vi "UpdateChanged.vi"(10 "WorldMapEdge":T1, 11 "RVCLibrary_Bug in":refnum<class "RVCLibrary_Bug2.lvclass">) -> (2 "updated":bool, 3 "RVCLibrary_Bug2 out":refnum<class "RVCLibrary_Bug2.lvclass">)   [LabVIEW 2013, in "RVCLibrary_Bug2.lvclass"]
uses:
  RVCLibrary_Bug2.lvclass
  <vilib>/robotics/Navigation/shared/MapNode/AbstractMapNode/NI_Robotics_AbstractMapNode.lvclass
  <vilib>/robotics/Navigation/shared/MapNode/AbstractDstarNode/NI_Robotics_AbstractDstarNode.lvclass
  <vilib>/robotics/Navigation/shared/WorldMap/World Map Edge.ctl
  <vilib>/robotics/Navigation/shared/WorldMap/AbstractWorldMap/NI_Robotics_AbstractWorldMap.lvclass
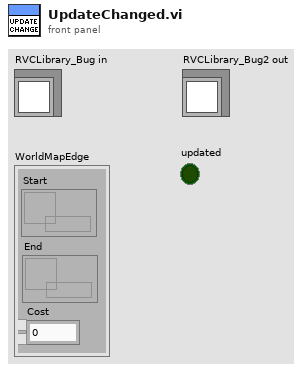
[diagram p1: front panel]
types:
  T1 = typedef "NI_Robotics_AbstractWorldMap.lvclass/World Map Edge.ctl" = cluster{"Start":refnum<data-value>, "End":refnum<data-value>, "Cost":dbl}
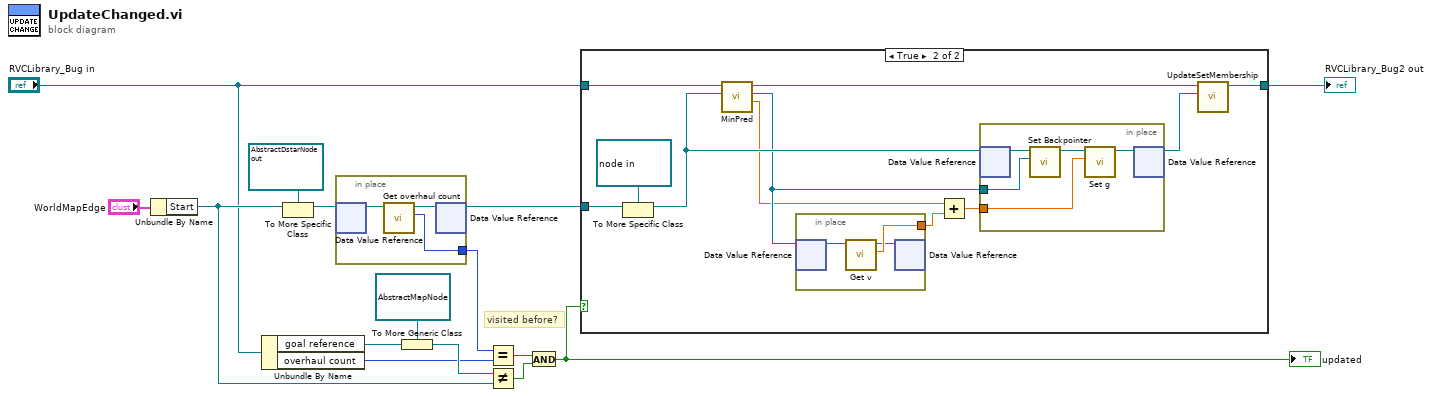
[diagram p0: block diagram]
diagram:
  # "visited before?"
  n1 = Unbundle By Name("WorldMapEdge") -> ("Start"=w10:refnum<data-value>)
  n2 = Unbundle By Name("RVCLibrary_Bug in") -> ("goal reference"=w9:refnum<data-value>, "overhaul count"=w7:i32)
  n3 = To More Specific Class(target class=refnum<data-value> refnum ("data value reference"), reference=w10) -> (specific class reference=w5:refnum<data-value>)  [unwired: 1 in, 1 out]
  n4 = in-place {
    in-place-border: [w18] -> w8
    n5 = in-place-dvr #1(w5) -> (w17:refnum<class "NI_Robotics_AbstractDstarNode.lvclass">)  [unwired: 1 out]
    n6 = call <vilib>:"Get overhaul count.vi"("AbstractDstarNode in"=w17) -> ("overhaul count"=w18:i32, "AbstractDstarNode out"=w16:refnum<class "NI_Robotics_AbstractDstarNode.lvclass">)  [unwired: 9 in]
    n7 = in-place-dvr #1(w16) -> (w4:refnum<data-value>)  [unwired: 1 out]
  }
  n8 = To More Generic Class(target class=refnum<data-value> refnum ("Start"), reference=w9) -> (generic class reference=w14:refnum<data-value>)
  n9 = Equal?(x=w8, y=w7) -> (x = y?=w6:bool)
  n10 = Not Equal?(x=w14, y=w10) -> (x != y?=w12:bool)
  n11 = And(x=w6, y=w12) -> (x .and. y?=w3:bool)
  "updated" <- w3
  n12 = case shown="True" w3 {
    tunnel: "RVCLibrary_Bug in" -> [w19 w20]
    tunnel: w4 -> [_ w25]
    tunnel: [w19 w27] -> w1
    frame False {
    }
    frame True {
      n13 = To More Specific Class(target class=refnum<data-value> refnum ("node ref in"), reference=w25) -> (specific class reference=w30:refnum<data-value>)  [unwired: 1 in, 1 out]
      n14 = call "MinPred.vi"("node ref in"=w30, "RVCLibrary_Bug in"=w20) -> ("cost of node to min pred"=w22:dbl, "min node ref"=w24:refnum<data-value>, "RVCLibrary_Bug out"=w28:refnum<class "RVCLibrary_Bug2.lvclass">)  [unwired: 6 in, 1 out]
      n15 = in-place {
        in-place-border: [w33] -> w23
        n16 = in-place-dvr #2(w24) -> (w32:refnum<class "NI_Robotics_AbstractDstarNode.lvclass">)  [unwired: 1 out]
        n17 = call <vilib>:"Get v.vi"("AbstractDstarNode in"=w32) -> ("v"=w33:dbl, "AbstractDstarNode out"=w31:refnum<class "NI_Robotics_AbstractDstarNode.lvclass">)  [unwired: 9 in]
        n18 = in-place-dvr #2(w31) -> ()  [unwired: 2 out]
      }
      n19 = Add(x=w22, y=w23) -> (x+y=w21:dbl)
      n20 = in-place {
        in-place-border: w24 -> [w38]
        in-place-border: w21 -> [w34]
        n21 = in-place-dvr #3(w30) -> (w37:refnum<class "NI_Robotics_AbstractDstarNode.lvclass">)  [unwired: 1 out]
        n22 = call <vilib>:"Set Backpointer.vi"("BackPointer"=w38, "AbstractDstarNode in"=w37) -> ("AbstractDstarNode out"=w36:refnum<class "NI_Robotics_AbstractDstarNode.lvclass">)  [unwired: 8 in, 1 out]
        n23 = call <vilib>:"Set g.vi"("g"=w34, "AbstractDstarNode in"=w36) -> ("AbstractDstarNode out"=w35:refnum<class "NI_Robotics_AbstractDstarNode.lvclass">)  [unwired: 9 in]
        n24 = in-place-dvr #3(w35) -> (w29:refnum<data-value>)  [unwired: 1 out]
      }
      n25 = call "UpdateSetMembership.vi"("node ref in"=w29, "RVCLibrary_Bug in"=w28) -> ("RVCLibrary_Bug out"=w27:refnum<class "RVCLibrary_Bug2.lvclass">)  [unwired: 8 in, 1 out]
    }
  }
  "RVCLibrary_Bug2 out" <- w1
